vi "RSZVB Trace Response Data.vi"(8 "error in (no error)":errorcluster {"code" format="%.0x"}, 9 "Data Format (0: Unformatted)":i32(ring) items=["Unformatted", "Formatted", "Unformatted With Trace Mathematics", "Pulse Profile"], 10 "Channel (Trace) (1)":i32=1, 11 "VISA session":refnum<visa-resource-name>) -> (0 "error out":errorcluster {"code" format="%.0x"}, 1 "Trace Data":dbl[](array[numeric]) format="%^.3e", 3 "dup VISA session":refnum<visa-resource-name>)   [LabVIEW 2015]
doc: "This VI reads the current response values of the active data trace or memory trace.\n\nRemote-control command(s):\nFORMat[:DATA] REAL ,32\nCALCulate<Ch/Tr>:DATA? FDATa | SDATa | MDATa | TSData"
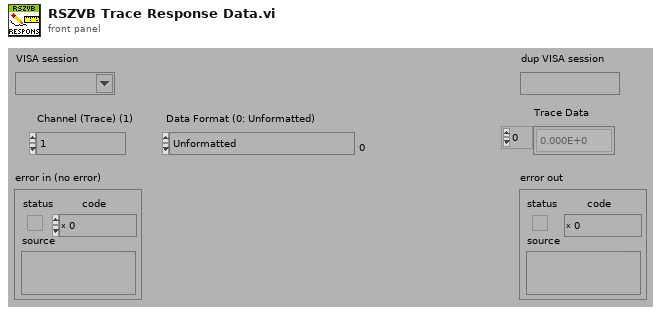
[diagram p1: front panel]
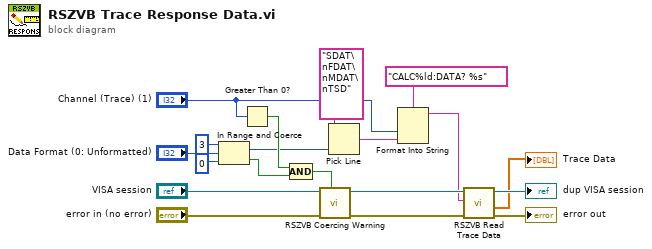
[diagram p0: block diagram]
diagram:
  n1 = In Range and Coerce(upper limit=3, x="Data Format (0: Unformatted)", lower limit=0) -> (coerced(x)=w4:i32, In Range?=w13:bool)
  n2 = Greater Than 0?(x="Channel (Trace) (1)") -> (x > 0?=w14:bool)
  n3 = Compound Arithmetic op=AND(w14, w13) -> (w15:bool)
  n4 = call "RSZVB Coercing Warning.vi"("In Range?"=w15, "error in (no error)"="error in (no error)", "VISA session"="VISA session") -> ("error out"=w12:errorcluster, "dup VISA session"=w11:refnum<visa-resource-name>)  [unwired: 7 in]
  n5 = Pick Line(multi-line string="SDAT\nFDAT\nMDAT\nTSD", line index=w4) -> (output string=w2:string)  [unwired: 1 in]
  n6 = Format Into String(format string="CALC%ld:DATA? %s", "Channel (Trace) (1)", w2) -> (resulting string=w1:string)  [unwired: 2 in, 1 out]
  n7 = call "RSZVB Read Trace Data.vi"("error in (no error)"=w12, "Buffer"=w1, "VISA session"=w11) -> ("error out"=→"error out":errorcluster, "Trace Data"=→"Trace Data":dbl[], "dup VISA session"=→"dup VISA session":refnum<visa-resource-name>)  [unwired: 6 in]
